vi "Default User Interface.vi"(8 "error in (no error)":errorcluster, 9 "index":i32, 10 "User Interface Events":refnum<class "User Interface Events.lvclass">, 11 "Configuration in":refnum<class "Configuration.lvclass">) -> (0 "error out":errorcluster, 3 "Configuration out":refnum<class "Configuration.lvclass">)   [LabVIEW 2017, in "DSF Core.lvlib" / "User Interface.lvclass"]
uses:
  User Interface.lvclass
  Configuration/Configuration.lvclass
  User Interface Events/User Interface Events.lvclass
panel:
  out "Data Version":string
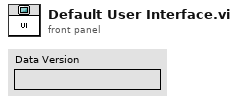
[diagram p1: front panel]
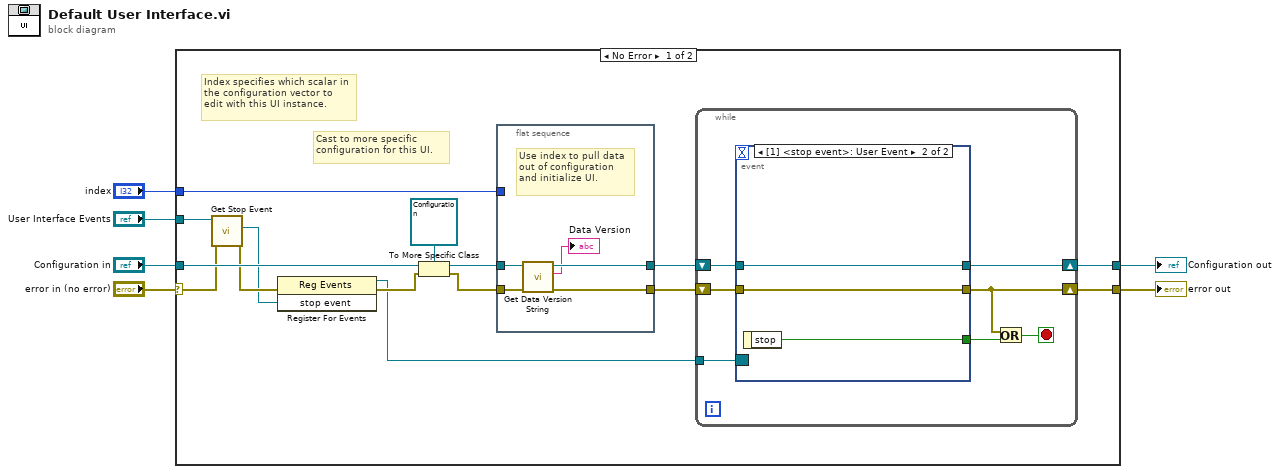
[diagram p0: block diagram]
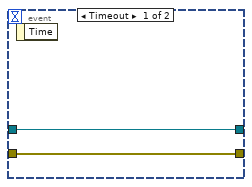
[diagram p2: hidden frame]
diagram:
  n1 = case shown="No Error" "error in (no error)" {
    selector: "error in (no error)" -> [w11 w40]
    tunnel: [w13 w40] -> w6
    tunnel: "index" -> [w17 _]
    tunnel: "Configuration in" -> [w16 w39]
    tunnel: [w14 w39] -> w2
    tunnel: "User Interface Events" -> [w12 _]
    frame No Error {
      # "Index specifies which scalar in the configuration vector to edit with this UI instance."
      # "Cast to more specific configuration for this UI."
      n2 = call "Get Stop Event.vi"("error in (no error)"=w11, "User Interface Events in"=w12) -> ("error out"=w10:errorcluster, "stop event"=w7:refnum<user-event>)  [unwired: 7 in, 1 out]
      n3 = register-events(error in=w10, w7) -> (reference out=w8:refnum<event-registration>, error out=w9:errorcluster)  [unwired: 1 in]
      n4 = To More Specific Class(target class=refnum<class "Configuration.lvclass"> refnum ("Configuration out"), reference=w16, error in=w9) -> (specific class reference=w21:refnum<class "Configuration.lvclass">, error out=w15:errorcluster)
      n5 = flat-sequence {
        tunnel: [w24] -> w18
        tunnel: w15 -> [w26]
        tunnel: w21 -> [w25]
        tunnel: [w23] -> w19
        tunnel: w17 -> [_]
        frame #0 {
          # "Use index to pull data out of configuration and initialize UI."
          n6 = call "Get Data Version String.vi"("error in (no error)"=w26, "Configuration in"=w25) -> ("error out"=w24:errorcluster, "data version"=→"Data Version":string, "Configuration out"=w23:refnum<class "Configuration.lvclass">)  [unwired: 7 in]
        }
      }
      n7 = while {
        tunnel: w8 -> [w33]
        shift-right: [w31] -> w13
        shift-left: w18 -> [w32]
        shift-right: [w27] -> w14
        shift-left: w19 -> [w28]
        stop <- w30 stop-if-true
        n8 = event shown="[1] <stop event>: User Event" {
          selector: w33 -> [_ _]
          dyn-events: _ -> [_ _]
          timeout: _ -> [_ _]
          tunnel: [_ w36] -> w29
          tunnel: w32 -> [w35 w38]
          tunnel: [w35 w38] -> w31
          tunnel: w28 -> [w34 w37]
          tunnel: [w34 w37] -> w27
          event Timeout {
            n9 = event-data() -> ()  [unwired: 1 in, 1 out]
          }
          event User Event {
            n10 = event-data() -> ("stop"=w36:bool)  [unwired: 1 in]
          }
        }
        n11 = Or(x=w31, y=w29) -> (x .or. y?=w30:bool)
      }
    }
    frame Error {
    }
  }
  "error out" <- w6
  "Configuration out" <- w2
